vi "PRL BUFFER Rearrange Timestamp Array.vi"(10 "Cut Index":i32, 11 "Array In":timestamp[](array[timestamp])) -> (3 "Array Out":timestamp[](array[timestamp]))   [LabVIEW 2017, in "PMU Recorder Light.lvlib"]
uses:
  PMU Recorder Light.lvlib
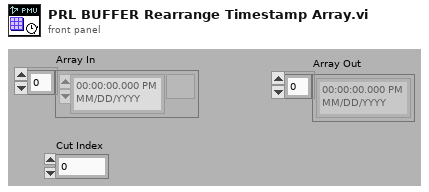
[diagram p1: front panel]
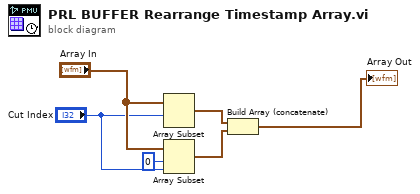
[diagram p0: block diagram]
diagram:
  n1 = Array Subset(array="Array In", index="Cut Index") -> (w3:timestamp[])  [unwired: 1 in]
  n2 = Array Subset(array="Array In", index=0, length="Cut Index") -> (w2:timestamp[])
  n3 = Build Array (concatenate)(w3, w2) -> (→"Array Out":timestamp[])
